vi "Visible_Ch_Init.vi"   [LabVIEW 2017]
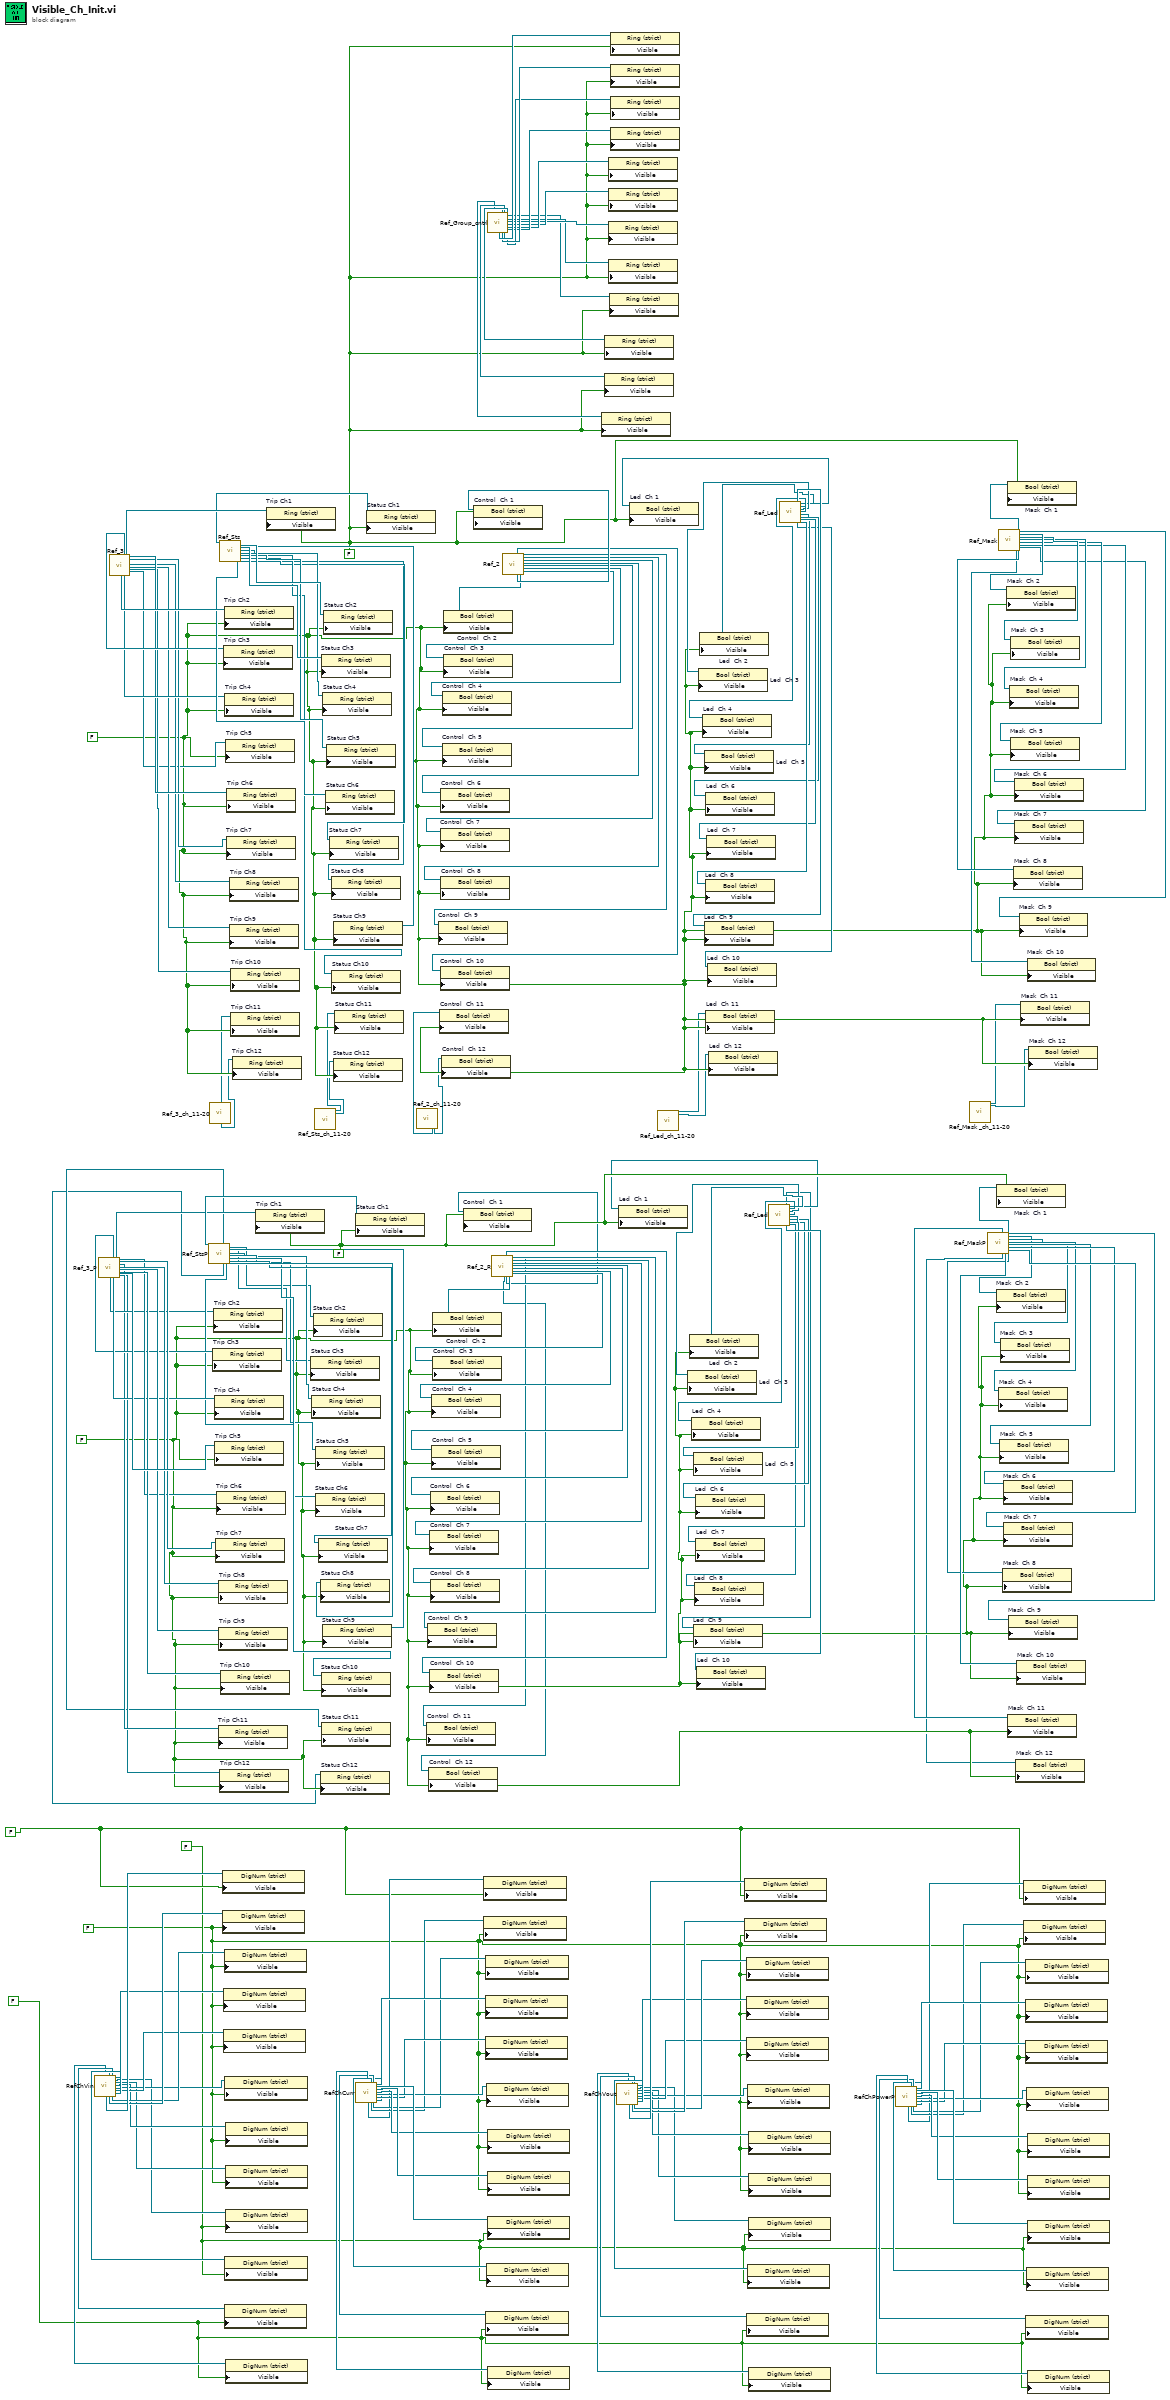
[diagram p0: block diagram]
diagram:
  w14 = FALSE
  w15 = FALSE
  w16 = FALSE
  w17 = FALSE
  w82 = FALSE
  w126 = FALSE
  w76 = FALSE
  w1 = FALSE
  n1 = call "RefChVin.vi"() -> ("Vin  P1 out"=w65:refnum<vi>, "Vin  P12 out"=w54:refnum<vi>, "Vin  P2 out"=w64:refnum<vi>, "Vin  P11 out"=w55:refnum<vi>, "Vin  P3 out"=w63:refnum<vi>, "Vin  P10 out"=w56:refnum<vi>, "Vin  P9 out"=w57:refnum<vi>, "Vin  P8 out"=w58:refnum<vi>, "Vin  P7 out"=w59:refnum<vi>, "Vin  P6 out"=w60:refnum<vi>, "Vin  P5 out"=w61:refnum<vi>, "Vin  P4 out"=w62:refnum<vi>)  [unwired: 15 in, 1 out]
  n2 = call "Ref_3_P.vi"() -> ("Trip  Ch 1 out"=w86:refnum<vi>, "Trip  Ch 2 out"=w89:refnum<vi>, "Trip  Ch 3 out"=w105:refnum<vi>, "Trip  Ch 4 out"=w106:refnum<vi>, "Trip  Ch 5 out"=w125:refnum<vi>, "Trip  Ch 6 out"=w107:refnum<vi>, "Trip  Ch 7 out"=w108:refnum<vi>, "Trip  Ch 11 out"=w85:refnum<vi>, "Trip  Ch 8 out"=w109:refnum<vi>, "Trip  Ch 9 out"=w110:refnum<vi>, "Trip  Ch 10 out"=w111:refnum<vi>, "Trip  Ch 12 out"=w84:refnum<vi>)  [unwired: 16 in]
  n3 = call "Ref_3.vi"() -> ("Trip  Ch 1 out"=w186:refnum<vi>, "Trip  Ch 2 out"=w183:refnum<vi>, "Trip  Ch 3 out"=w167:refnum<vi>, "Trip  Ch 4 out"=w166:refnum<vi>, "Trip  Ch 5 out"=w147:refnum<vi>, "Trip  Ch 6 out"=w165:refnum<vi>, "Trip  Ch 7 out"=w164:refnum<vi>, "Trip  Ch 8 out"=w163:refnum<vi>, "Trip  Ch 9 out"=w162:refnum<vi>, "Trip  Ch 10 out"=w161:refnum<vi>)  [unwired: 18 in]
  n4 = call "Ref_StsP.vi"() -> ("Status Ch11 out"=w83:refnum<vi>, "Status Ch12 out"=w81:refnum<vi>, "Status Ch9 out"=w103:refnum<vi>, "Status Ch10 out"=w104:refnum<vi>, "Status Ch1 out"=w87:refnum<vi>, "Status Ch2 out"=w97:refnum<vi>, "Status Ch3 out"=w98:refnum<vi>, "Status Ch4 out"=w99:refnum<vi>, "Status Ch5 out"=w100:refnum<vi>, "Status Ch6 out"=w101:refnum<vi>, "Status Ch7 out"=w102:refnum<vi>, "Status Ch8 out"=w114:refnum<vi>)  [unwired: 16 in]
  n5 = call "Ref_3_ch_11-20.vi"() -> ("Trip  Ch 11 out"=w75:refnum<vi>, "Trip  Ch 12 out"=w74:refnum<vi>)  [unwired: 18 in, 8 out]
  n6 = property on="Trip Ch3" class="Ring (strict)"(reference=w105, "Visible"=w82) -> ()  [unwired: 1 in, 2 out]
  n7 = property on="Trip Ch2" class="Ring (strict)"(reference=w89, "Visible"=w82) -> ()  [unwired: 1 in, 2 out]
  n8 = property on="Trip Ch4" class="Ring (strict)"(reference=w106, "Visible"=w82) -> ()  [unwired: 1 in, 2 out]
  n9 = property on="Trip Ch5" class="Ring (strict)"(reference=w125, "Visible"=w82) -> ()  [unwired: 1 in, 2 out]
  n10 = property on="Trip Ch7" class="Ring (strict)"(reference=w108, "Visible"=w82) -> ()  [unwired: 1 in, 2 out]
  n11 = property on="Trip Ch6" class="Ring (strict)"(reference=w107, "Visible"=w82) -> ()  [unwired: 1 in, 2 out]
  n12 = property on="Trip Ch11" class="Ring (strict)"(reference=w85, "Visible"=w82) -> ()  [unwired: 1 in, 2 out]
  n13 = property on="Trip Ch8" class="Ring (strict)"(reference=w109, "Visible"=w82) -> ()  [unwired: 1 in, 2 out]
  n14 = property on="Trip Ch9" class="Ring (strict)"(reference=w110, "Visible"=w82) -> ()  [unwired: 1 in, 2 out]
  n15 = call "Ref_Sts.vi"() -> ("Status Ch9 out"=w169:refnum<vi>, "Status Ch10 out"=w168:refnum<vi>, "Status Ch1 out"=w185:refnum<vi>, "Status Ch2 out"=w175:refnum<vi>, "Status Ch3 out"=w174:refnum<vi>, "Status Ch4 out"=w173:refnum<vi>, "Status Ch5 out"=w172:refnum<vi>, "Status Ch6 out"=w171:refnum<vi>, "Status Ch7 out"=w170:refnum<vi>, "Status Ch8 out"=w158:refnum<vi>)  [unwired: 18 in]
  n16 = property on="Trip Ch12" class="Ring (strict)"(reference=w84, "Visible"=w82) -> ()  [unwired: 1 in, 2 out]
  n17 = property on="Trip Ch10" class="Ring (strict)"(reference=w111, "Visible"=w82) -> ()  [unwired: 1 in, 2 out]
  n18 = property class="DigNum (strict)"(reference=w65, "Visible"=w16) -> ()  [unwired: 1 in, 2 out]
  n19 = property class="DigNum (strict)"(reference=w64, "Visible"=w14) -> ()  [unwired: 1 in, 2 out]
  n20 = property on="Trip Ch3" class="Ring (strict)"(reference=w167, "Visible"=w76) -> ()  [unwired: 1 in, 2 out]
  n21 = property class="DigNum (strict)"(reference=w62, "Visible"=w14) -> ()  [unwired: 1 in, 2 out]
  n22 = property class="DigNum (strict)"(reference=w61, "Visible"=w14) -> ()  [unwired: 1 in, 2 out]
  n23 = property on="Trip Ch2" class="Ring (strict)"(reference=w183, "Visible"=w76) -> ()  [unwired: 1 in, 2 out]
  n24 = property class="DigNum (strict)"(reference=w63, "Visible"=w14) -> ()  [unwired: 1 in, 2 out]
  n25 = property class="DigNum (strict)"(reference=w55, "Visible"=w17) -> ()  [unwired: 1 in, 2 out]
  n26 = property on="Trip Ch4" class="Ring (strict)"(reference=w166, "Visible"=w76) -> ()  [unwired: 1 in, 2 out]
  n27 = property class="DigNum (strict)"(reference=w60, "Visible"=w14) -> ()  [unwired: 1 in, 2 out]
  n28 = property class="DigNum (strict)"(reference=w56, "Visible"=w15) -> ()  [unwired: 1 in, 2 out]
  n29 = property on="Trip Ch5" class="Ring (strict)"(reference=w147, "Visible"=w76) -> ()  [unwired: 1 in, 2 out]
  n30 = property class="DigNum (strict)"(reference=w59, "Visible"=w14) -> ()  [unwired: 1 in, 2 out]
  n31 = property class="DigNum (strict)"(reference=w58, "Visible"=w14) -> ()  [unwired: 1 in, 2 out]
  n32 = property class="DigNum (strict)"(reference=w57, "Visible"=w15) -> ()  [unwired: 1 in, 2 out]
  n33 = property class="DigNum (strict)"(reference=w54, "Visible"=w17) -> ()  [unwired: 1 in, 2 out]
  n34 = property on="Trip Ch7" class="Ring (strict)"(reference=w164, "Visible"=w76) -> ()  [unwired: 1 in, 2 out]
  n35 = property on="Trip Ch6" class="Ring (strict)"(reference=w165, "Visible"=w76) -> ()  [unwired: 1 in, 2 out]
  n36 = property on="Trip Ch8" class="Ring (strict)"(reference=w163, "Visible"=w76) -> ()  [unwired: 1 in, 2 out]
  n37 = property on="Trip Ch9" class="Ring (strict)"(reference=w162, "Visible"=w76) -> ()  [unwired: 1 in, 2 out]
  n38 = property on="Trip Ch10" class="Ring (strict)"(reference=w161, "Visible"=w76) -> ()  [unwired: 1 in, 2 out]
  n39 = property on="Trip Ch11" class="Ring (strict)"(reference=w75, "Visible"=w76) -> ()  [unwired: 1 in, 2 out]
  n40 = property on="Trip Ch12" class="Ring (strict)"(reference=w74, "Visible"=w76) -> ()  [unwired: 1 in, 2 out]
  n41 = property on="Trip Ch1" class="Ring (strict)"(reference=w86, "Visible"=w126) -> ()  [unwired: 1 in, 2 out]
  n42 = property on="Trip Ch1" class="Ring (strict)"(reference=w186, "Visible"=w1) -> ()  [unwired: 1 in, 2 out]
  n43 = property on="Status Ch3" class="Ring (strict)"(reference=w98, "Visible"=w82) -> ()  [unwired: 1 in, 2 out]
  n44 = property on="Status Ch4" class="Ring (strict)"(reference=w99, "Visible"=w82) -> ()  [unwired: 1 in, 2 out]
  n45 = property on="Status Ch2" class="Ring (strict)"(reference=w97, "Visible"=w82) -> ()  [unwired: 1 in, 2 out]
  n46 = call "Ref_Sts_ch_11-20.vi"() -> ("Status Ch 11 out"=w73:refnum<vi>, "Status Ch 12 out"=w72:refnum<vi>)  [unwired: 18 in, 8 out]
  n47 = property on="Status Ch6" class="Ring (strict)"(reference=w101, "Visible"=w82) -> ()  [unwired: 1 in, 2 out]
  n48 = property on="Status Ch5" class="Ring (strict)"(reference=w100, "Visible"=w82) -> ()  [unwired: 1 in, 2 out]
  n49 = property on="Status Ch7" class="Ring (strict)"(reference=w102, "Visible"=w82) -> ()  [unwired: 1 in, 2 out]
  n50 = property on="Status Ch8" class="Ring (strict)"(reference=w114, "Visible"=w82) -> ()  [unwired: 1 in, 2 out]
  n51 = property on="Status Ch12" class="Ring (strict)"(reference=w81, "Visible"=w82) -> ()  [unwired: 1 in, 2 out]
  n52 = property on="Status Ch3" class="Ring (strict)"(reference=w174, "Visible"=w76) -> ()  [unwired: 1 in, 2 out]
  n53 = property on="Status Ch10" class="Ring (strict)"(reference=w104, "Visible"=w82) -> ()  [unwired: 1 in, 2 out]
  n54 = property on="Status Ch11" class="Ring (strict)"(reference=w83, "Visible"=w82) -> ()  [unwired: 1 in, 2 out]
  n55 = property on="Status Ch4" class="Ring (strict)"(reference=w173, "Visible"=w76) -> ()  [unwired: 1 in, 2 out]
  n56 = property on="Status Ch9" class="Ring (strict)"(reference=w103, "Visible"=w82) -> ()  [unwired: 1 in, 2 out]
  n57 = property on="Status Ch2" class="Ring (strict)"(reference=w175, "Visible"=w76) -> ()  [unwired: 1 in, 2 out]
  n58 = property on="Status Ch6" class="Ring (strict)"(reference=w171, "Visible"=w76) -> ()  [unwired: 1 in, 2 out]
  n59 = property on="Status Ch5" class="Ring (strict)"(reference=w172, "Visible"=w76) -> ()  [unwired: 1 in, 2 out]
  n60 = property on="Status Ch7" class="Ring (strict)"(reference=w170, "Visible"=w76) -> ()  [unwired: 1 in, 2 out]
  n61 = property on="Status Ch8" class="Ring (strict)"(reference=w158, "Visible"=w76) -> ()  [unwired: 1 in, 2 out]
  n62 = property on="Status Ch10" class="Ring (strict)"(reference=w168, "Visible"=w76) -> ()  [unwired: 1 in, 2 out]
  n63 = property on="Status Ch9" class="Ring (strict)"(reference=w169, "Visible"=w76) -> ()  [unwired: 1 in, 2 out]
  n64 = property on="Status Ch12" class="Ring (strict)"(reference=w72, "Visible"=w76) -> ()  [unwired: 1 in, 2 out]
  n65 = property on="Status Ch11" class="Ring (strict)"(reference=w73, "Visible"=w76) -> ()  [unwired: 1 in, 2 out]
  n66 = property on="Status Ch1" class="Ring (strict)"(reference=w87, "Visible"=w126) -> ()  [unwired: 1 in, 2 out]
  n67 = call "RefChCurr.vi"() -> ("Current P1 out"=w42:refnum<vi>, "Current P12 out"=w53:refnum<vi>, "Current P2 out"=w43:refnum<vi>, "Current P11 out"=w52:refnum<vi>, "Current P3 out"=w44:refnum<vi>, "Current P10 out"=w51:refnum<vi>, "Current P9 out"=w50:refnum<vi>, "Current P8 out"=w49:refnum<vi>, "Current P7 out"=w48:refnum<vi>, "Current P6 out"=w47:refnum<vi>, "Current P5 out"=w46:refnum<vi>, "Current P4 out"=w45:refnum<vi>)  [unwired: 15 in, 1 out]
  n68 = property on="Status Ch1" class="Ring (strict)"(reference=w185, "Visible"=w1) -> ()  [unwired: 1 in, 2 out]
  n69 = call "Ref_2_ch_11-20.vi"() -> ("Control  Ch 11 out"=w71:refnum<vi>, "Control  Ch 12 out"=w70:refnum<vi>)  [unwired: 17 in, 9 out]
  n70 = property on="Control  Ch 11" class="Bool (strict)"(reference=w71, "Visible"=w76) -> ()  [unwired: 1 in, 2 out]
  n71 = property on="Control  Ch 12" class="Bool (strict)"(reference=w70, "Visible"=w76) -> ()  [unwired: 1 in, 2 out]
  n72 = property class="DigNum (strict)"(reference=w42, "Visible"=w16) -> ()  [unwired: 1 in, 2 out]
  n73 = property class="DigNum (strict)"(reference=w43, "Visible"=w14) -> ()  [unwired: 1 in, 2 out]
  n74 = property class="DigNum (strict)"(reference=w45, "Visible"=w14) -> ()  [unwired: 1 in, 2 out]
  n75 = property class="DigNum (strict)"(reference=w46, "Visible"=w14) -> ()  [unwired: 1 in, 2 out]
  n76 = property class="DigNum (strict)"(reference=w44, "Visible"=w14) -> ()  [unwired: 1 in, 2 out]
  n77 = property class="DigNum (strict)"(reference=w52, "Visible"=w17) -> ()  [unwired: 1 in, 2 out]
  n78 = property class="DigNum (strict)"(reference=w47, "Visible"=w14) -> ()  [unwired: 1 in, 2 out]
  n79 = property class="DigNum (strict)"(reference=w51, "Visible"=w15) -> ()  [unwired: 1 in, 2 out]
  n80 = call "Ref_Group_cntrl.vi"() -> ("Group ch 1 out"=w13:refnum<vi>, "Group ch 12 out"=w2:refnum<vi>, "Group ch 2 out"=w12:refnum<vi>, "Group ch 11 out"=w3:refnum<vi>, "Group ch 3 out"=w11:refnum<vi>, "Group ch 10 out"=w4:refnum<vi>, "Group ch 9 out"=w5:refnum<vi>, "Group ch 8 out"=w6:refnum<vi>, "Group ch 7 out"=w7:refnum<vi>, "Group ch 6 out"=w8:refnum<vi>, "Group ch 5 out"=w9:refnum<vi>, "Group ch 4 out"=w10:refnum<vi>)  [unwired: 15 in, 1 out]
  n81 = property class="DigNum (strict)"(reference=w48, "Visible"=w14) -> ()  [unwired: 1 in, 2 out]
  n82 = property class="DigNum (strict)"(reference=w49, "Visible"=w14) -> ()  [unwired: 1 in, 2 out]
  n83 = property class="DigNum (strict)"(reference=w50, "Visible"=w15) -> ()  [unwired: 1 in, 2 out]
  n84 = property class="DigNum (strict)"(reference=w53, "Visible"=w17) -> ()  [unwired: 1 in, 2 out]
  n85 = call "Ref_2_R.vi"() -> ("Control  Ch 12 out"=w79:refnum<vi>, "Control  Ch 10 out"=w96:refnum<vi>, "Control  Ch 1 out"=w88:refnum<vi>, "Control  Ch 9 out"=w95:refnum<vi>, "Control  Ch 2 out"=w90:refnum<vi>, "Control  Ch 11 out"=w80:refnum<vi>, "Control  Ch 8 out"=w94:refnum<vi>, "Control  Ch 7 out"=w93:refnum<vi>, "Control  Ch 6 out"=w113:refnum<vi>, "Control  Ch 5 out"=w92:refnum<vi>, "Control  Ch 4 out"=w91:refnum<vi>, "Control  Ch 3 out"=w112:refnum<vi>)  [unwired: 15 in, 1 out]
  n86 = property on="Control  Ch 11" class="Bool (strict)"(reference=w80, "Visible"=w82) -> ()  [unwired: 1 in, 2 out]
  n87 = property on="Control  Ch 9" class="Bool (strict)"(reference=w95, "Visible"=w82) -> ()  [unwired: 1 in, 2 out]
  n88 = property on="Control  Ch 12" class="Bool (strict)"(reference=w79, "Visible"=w82) -> ()  [unwired: 1 in, 2 out]
  n89 = property on="Control  Ch 7" class="Bool (strict)"(reference=w93, "Visible"=w82) -> ()  [unwired: 1 in, 2 out]
  n90 = property on="Control  Ch 10" class="Bool (strict)"(reference=w96, "Visible"=w82) -> ()  [unwired: 1 in, 2 out]
  n91 = property on="Control  Ch 6" class="Bool (strict)"(reference=w113, "Visible"=w82) -> ()  [unwired: 1 in, 2 out]
  n92 = property on="Control  Ch 8" class="Bool (strict)"(reference=w94, "Visible"=w82) -> ()  [unwired: 1 in, 2 out]
  n93 = property on="Control  Ch 4" class="Bool (strict)"(reference=w91, "Visible"=w82) -> ()  [unwired: 1 in, 2 out]
  n94 = property on="Control  Ch 5" class="Bool (strict)"(reference=w92, "Visible"=w82) -> ()  [unwired: 1 in, 2 out]
  n95 = property on="Control  Ch 2" class="Bool (strict)"(reference=w90, "Visible"=w82) -> ()  [unwired: 1 in, 2 out]
  n96 = property on="Control  Ch 3" class="Bool (strict)"(reference=w112, "Visible"=w82) -> ()  [unwired: 1 in, 2 out]
  n97 = property on="Control  Ch 1" class="Bool (strict)"(reference=w88, "Visible"=w126) -> ()  [unwired: 1 in, 2 out]
  n98 = call "Ref_2.vi"() -> ("Control  Ch 10 out"=w176:refnum<vi>, "Control  Ch 1 out"=w184:refnum<vi>, "Control  Ch 9 out"=w177:refnum<vi>, "Control  Ch 2 out"=w182:refnum<vi>, "Control  Ch 8 out"=w178:refnum<vi>, "Control  Ch 7 out"=w179:refnum<vi>, "Control  Ch 6 out"=w159:refnum<vi>, "Control  Ch 5 out"=w180:refnum<vi>, "Control  Ch 4 out"=w181:refnum<vi>, "Control  Ch 3 out"=w160:refnum<vi>)  [unwired: 17 in, 1 out]
  n99 = property on="Control  Ch 9" class="Bool (strict)"(reference=w177, "Visible"=w76) -> ()  [unwired: 1 in, 2 out]
  n100 = property on="Control  Ch 7" class="Bool (strict)"(reference=w179, "Visible"=w76) -> ()  [unwired: 1 in, 2 out]
  n101 = property on="Control  Ch 10" class="Bool (strict)"(reference=w176, "Visible"=w76) -> ()  [unwired: 1 in, 2 out]
  n102 = property on="Control  Ch 6" class="Bool (strict)"(reference=w159, "Visible"=w76) -> ()  [unwired: 1 in, 2 out]
  n103 = property on="Control  Ch 8" class="Bool (strict)"(reference=w178, "Visible"=w76) -> ()  [unwired: 1 in, 2 out]
  n104 = property on="Control  Ch 4" class="Bool (strict)"(reference=w181, "Visible"=w76) -> ()  [unwired: 1 in, 2 out]
  n105 = property on="Control  Ch 5" class="Bool (strict)"(reference=w180, "Visible"=w76) -> ()  [unwired: 1 in, 2 out]
  n106 = property on="Control  Ch 2" class="Bool (strict)"(reference=w182, "Visible"=w76) -> ()  [unwired: 1 in, 2 out]
  n107 = property on="Control  Ch 3" class="Bool (strict)"(reference=w160, "Visible"=w76) -> ()  [unwired: 1 in, 2 out]
  n108 = property on="Control  Ch 1" class="Bool (strict)"(reference=w184, "Visible"=w1) -> ()  [unwired: 1 in, 2 out]
  n109 = property class="Ring (strict)"(reference=w2, "Visible"=w1) -> ()  [unwired: 1 in, 2 out]
  n110 = property class="Ring (strict)"(reference=w3, "Visible"=w1) -> ()  [unwired: 1 in, 2 out]
  n111 = property class="Ring (strict)"(reference=w4, "Visible"=w1) -> ()  [unwired: 1 in, 2 out]
  n112 = property class="Ring (strict)"(reference=w7, "Visible"=w1) -> ()  [unwired: 1 in, 2 out]
  n113 = property class="Ring (strict)"(reference=w9, "Visible"=w1) -> ()  [unwired: 1 in, 2 out]
  n114 = property class="Ring (strict)"(reference=w8, "Visible"=w1) -> ()  [unwired: 1 in, 2 out]
  n115 = property class="Ring (strict)"(reference=w6, "Visible"=w1) -> ()  [unwired: 1 in, 2 out]
  n116 = property class="Ring (strict)"(reference=w5, "Visible"=w1) -> ()  [unwired: 1 in, 2 out]
  n117 = property class="Ring (strict)"(reference=w12, "Visible"=w1) -> ()  [unwired: 1 in, 2 out]
  n118 = property class="Ring (strict)"(reference=w10, "Visible"=w1) -> ()  [unwired: 1 in, 2 out]
  n119 = property class="Ring (strict)"(reference=w13, "Visible"=w1) -> ()  [unwired: 1 in, 2 out]
  n120 = property class="Ring (strict)"(reference=w11, "Visible"=w1) -> ()  [unwired: 1 in, 2 out]
  n121 = call "RefChVout.vi"() -> ("Vout  P1 out"=w41:refnum<vi>, "Vout  P12 out"=w30:refnum<vi>, "Vout  P2 out"=w40:refnum<vi>, "Vout  P11 out"=w31:refnum<vi>, "Vout  P3 out"=w39:refnum<vi>, "Vout  P10 out"=w32:refnum<vi>, "Vout  P9 out"=w33:refnum<vi>, "Vout  P8 out"=w34:refnum<vi>, "Vout  P7 out"=w35:refnum<vi>, "Vout  P6 out"=w36:refnum<vi>, "Vout  P5 out"=w37:refnum<vi>, "Vout  P4 out"=w38:refnum<vi>)  [unwired: 15 in, 1 out]
  n122 = call "Ref_Led_ch_11-20.vi"() -> ("Led Ch 11 out"=w69:refnum<vi>, "Led Ch 12 out"=w68:refnum<vi>)  [unwired: 18 in, 8 out]
  n123 = property on="Led  Ch 11" class="Bool (strict)"(reference=w69, "Visible"=w76) -> ()  [unwired: 1 in, 2 out]
  n124 = property on="Led  Ch 12" class="Bool (strict)"(reference=w68, "Visible"=w76) -> ()  [unwired: 1 in, 2 out]
  n125 = property class="DigNum (strict)"(reference=w41, "Visible"=w16) -> ()  [unwired: 1 in, 2 out]
  n126 = property class="DigNum (strict)"(reference=w40, "Visible"=w14) -> ()  [unwired: 1 in, 2 out]
  n127 = property class="DigNum (strict)"(reference=w38, "Visible"=w14) -> ()  [unwired: 1 in, 2 out]
  n128 = property class="DigNum (strict)"(reference=w37, "Visible"=w14) -> ()  [unwired: 1 in, 2 out]
  n129 = property class="DigNum (strict)"(reference=w39, "Visible"=w14) -> ()  [unwired: 1 in, 2 out]
  n130 = property class="DigNum (strict)"(reference=w31, "Visible"=w17) -> ()  [unwired: 1 in, 2 out]
  n131 = property class="DigNum (strict)"(reference=w36, "Visible"=w14) -> ()  [unwired: 1 in, 2 out]
  n132 = property class="DigNum (strict)"(reference=w32, "Visible"=w15) -> ()  [unwired: 1 in, 2 out]
  n133 = property class="DigNum (strict)"(reference=w35, "Visible"=w14) -> ()  [unwired: 1 in, 2 out]
  n134 = property class="DigNum (strict)"(reference=w34, "Visible"=w14) -> ()  [unwired: 1 in, 2 out]
  n135 = property class="DigNum (strict)"(reference=w33, "Visible"=w15) -> ()  [unwired: 1 in, 2 out]
  n136 = property class="DigNum (strict)"(reference=w30, "Visible"=w17) -> ()  [unwired: 1 in, 2 out]
  n137 = call "Ref_Led.vi"() -> ("Led Ch 9 out"=w115:refnum<vi>, "Led Ch 10 out"=w122:refnum<vi>, "Led Ch 1 out"=w123:refnum<vi>, "Led Ch 2 out"=w124:refnum<vi>, "Led Ch 3 out"=w121:refnum<vi>, "Led Ch 4 out"=w120:refnum<vi>, "Led Ch 5 out"=w119:refnum<vi>, "Led Ch 6 out"=w118:refnum<vi>, "Led Ch 7 out"=w117:refnum<vi>, "Led Ch 8 out"=w116:refnum<vi>)  [unwired: 18 in]
  n138 = property on="Led  Ch 1" class="Bool (strict)"(reference=w123, "Visible"=w126) -> ()  [unwired: 1 in, 2 out]
  n139 = property on="Led  Ch 3" class="Bool (strict)"(reference=w121, "Visible"=w82) -> ()  [unwired: 1 in, 2 out]
  n140 = property on="Led  Ch 2" class="Bool (strict)"(reference=w124, "Visible"=w82) -> ()  [unwired: 1 in, 2 out]
  n141 = property on="Led  Ch 4" class="Bool (strict)"(reference=w120, "Visible"=w82) -> ()  [unwired: 1 in, 2 out]
  n142 = property on="Led  Ch 5" class="Bool (strict)"(reference=w119, "Visible"=w82) -> ()  [unwired: 1 in, 2 out]
  n143 = property on="Led  Ch 9" class="Bool (strict)"(reference=w115, "Visible"=w82) -> ()  [unwired: 1 in, 2 out]
  n144 = property on="Led  Ch 8" class="Bool (strict)"(reference=w116, "Visible"=w82) -> ()  [unwired: 1 in, 2 out]
  n145 = property on="Led  Ch 6" class="Bool (strict)"(reference=w118, "Visible"=w82) -> ()  [unwired: 1 in, 2 out]
  n146 = property on="Led  Ch 7" class="Bool (strict)"(reference=w117, "Visible"=w82) -> ()  [unwired: 1 in, 2 out]
  n147 = property on="Led  Ch 10" class="Bool (strict)"(reference=w122, "Visible"=w82) -> ()  [unwired: 1 in, 2 out]
  n148 = call "Ref_Led.vi"() -> ("Led Ch 9 out"=w157:refnum<vi>, "Led Ch 10 out"=w150:refnum<vi>, "Led Ch 1 out"=w149:refnum<vi>, "Led Ch 2 out"=w148:refnum<vi>, "Led Ch 3 out"=w151:refnum<vi>, "Led Ch 4 out"=w152:refnum<vi>, "Led Ch 5 out"=w153:refnum<vi>, "Led Ch 6 out"=w154:refnum<vi>, "Led Ch 7 out"=w155:refnum<vi>, "Led Ch 8 out"=w156:refnum<vi>)  [unwired: 18 in]
  n149 = property on="Led  Ch 1" class="Bool (strict)"(reference=w149, "Visible"=w1) -> ()  [unwired: 1 in, 2 out]
  n150 = property on="Led  Ch 3" class="Bool (strict)"(reference=w151, "Visible"=w76) -> ()  [unwired: 1 in, 2 out]
  n151 = property on="Led  Ch 2" class="Bool (strict)"(reference=w148, "Visible"=w76) -> ()  [unwired: 1 in, 2 out]
  n152 = property on="Led  Ch 4" class="Bool (strict)"(reference=w152, "Visible"=w76) -> ()  [unwired: 1 in, 2 out]
  n153 = property on="Led  Ch 5" class="Bool (strict)"(reference=w153, "Visible"=w76) -> ()  [unwired: 1 in, 2 out]
  n154 = property on="Led  Ch 9" class="Bool (strict)"(reference=w157, "Visible"=w76) -> ()  [unwired: 1 in, 2 out]
  n155 = property on="Led  Ch 8" class="Bool (strict)"(reference=w156, "Visible"=w76) -> ()  [unwired: 1 in, 2 out]
  n156 = property on="Led  Ch 6" class="Bool (strict)"(reference=w154, "Visible"=w76) -> ()  [unwired: 1 in, 2 out]
  n157 = property on="Led  Ch 7" class="Bool (strict)"(reference=w155, "Visible"=w76) -> ()  [unwired: 1 in, 2 out]
  n158 = property on="Led  Ch 10" class="Bool (strict)"(reference=w150, "Visible"=w76) -> ()  [unwired: 1 in, 2 out]
  n159 = call "RefChPowerP.vi"() -> ("Pwr  P1 out"=w18:refnum<vi>, "Pwr  P12 out"=w29:refnum<vi>, "Pwr  P2 out"=w19:refnum<vi>, "Pwr  P11 out"=w28:refnum<vi>, "Pwr  P3 out"=w20:refnum<vi>, "Pwr  P10 out"=w27:refnum<vi>, "Pwr  P9 out"=w26:refnum<vi>, "Pwr  P8 out"=w25:refnum<vi>, "Pwr  P7 out"=w24:refnum<vi>, "Pwr  P6 out"=w23:refnum<vi>, "Pwr  P5 out"=w22:refnum<vi>, "Pwr  P4 out"=w21:refnum<vi>)  [unwired: 15 in, 1 out]
  n160 = call "Ref_Mask _ch_11-20.vi"() -> ("Mask Ch 11 out"=w67:refnum<vi>, "Mask Ch 12 out"=w66:refnum<vi>)  [unwired: 18 in, 8 out]
  n161 = call "Ref_MaskP.vi"() -> ("Mask Ch 11 out"=w78:refnum<vi>, "Mask Ch 12 out"=w77:refnum<vi>, "Mask Ch 9 out"=w136:refnum<vi>, "Mask Ch 10 out"=w134:refnum<vi>, "Mask Ch 1 out"=w135:refnum<vi>, "Mask Ch 2 out"=w127:refnum<vi>, "Mask Ch 3 out"=w128:refnum<vi>, "Mask Ch 4 out"=w129:refnum<vi>, "Mask Ch 5 out"=w130:refnum<vi>, "Mask Ch 6 out"=w131:refnum<vi>, "Mask Ch 7 out"=w132:refnum<vi>, "Mask Ch 8 out"=w133:refnum<vi>)  [unwired: 16 in]
  n162 = property on="Mask  Ch 2" class="Bool (strict)"(reference=w127, "Visible"=w82) -> ()  [unwired: 1 in, 2 out]
  n163 = property on="Mask  Ch 1" class="Bool (strict)"(reference=w135, "Visible"=w126) -> ()  [unwired: 1 in, 2 out]
  n164 = call "Ref_Mask.vi"() -> ("Mask Ch 9 out"=w137:refnum<vi>, "Mask Ch 10 out"=w139:refnum<vi>, "Mask Ch 1 out"=w138:refnum<vi>, "Mask Ch 2 out"=w146:refnum<vi>, "Mask Ch 3 out"=w145:refnum<vi>, "Mask Ch 4 out"=w144:refnum<vi>, "Mask Ch 5 out"=w143:refnum<vi>, "Mask Ch 6 out"=w142:refnum<vi>, "Mask Ch 7 out"=w141:refnum<vi>, "Mask Ch 8 out"=w140:refnum<vi>)  [unwired: 18 in]
  n165 = property on="Mask  Ch 4" class="Bool (strict)"(reference=w129, "Visible"=w82) -> ()  [unwired: 1 in, 2 out]
  n166 = property on="Mask  Ch 5" class="Bool (strict)"(reference=w130, "Visible"=w82) -> ()  [unwired: 1 in, 2 out]
  n167 = property on="Mask  Ch 3" class="Bool (strict)"(reference=w128, "Visible"=w82) -> ()  [unwired: 1 in, 2 out]
  n168 = property on="Mask  Ch 8" class="Bool (strict)"(reference=w133, "Visible"=w82) -> ()  [unwired: 1 in, 2 out]
  n169 = property on="Mask  Ch 6" class="Bool (strict)"(reference=w131, "Visible"=w82) -> ()  [unwired: 1 in, 2 out]
  n170 = property on="Mask  Ch 7" class="Bool (strict)"(reference=w132, "Visible"=w82) -> ()  [unwired: 1 in, 2 out]
  n171 = property on="Mask  Ch 2" class="Bool (strict)"(reference=w146, "Visible"=w76) -> ()  [unwired: 1 in, 2 out]
  n172 = property on="Mask  Ch 1" class="Bool (strict)"(reference=w138, "Visible"=w1) -> ()  [unwired: 1 in, 2 out]
  n173 = property on="Mask  Ch 11" class="Bool (strict)"(reference=w78, "Visible"=w82) -> ()  [unwired: 1 in, 2 out]
  n174 = property on="Mask  Ch 9" class="Bool (strict)"(reference=w136, "Visible"=w82) -> ()  [unwired: 1 in, 2 out]
  n175 = property on="Mask  Ch 4" class="Bool (strict)"(reference=w144, "Visible"=w76) -> ()  [unwired: 1 in, 2 out]
  n176 = property on="Mask  Ch 5" class="Bool (strict)"(reference=w143, "Visible"=w76) -> ()  [unwired: 1 in, 2 out]
  n177 = property on="Mask  Ch 3" class="Bool (strict)"(reference=w145, "Visible"=w76) -> ()  [unwired: 1 in, 2 out]
  n178 = property on="Mask  Ch 8" class="Bool (strict)"(reference=w140, "Visible"=w76) -> ()  [unwired: 1 in, 2 out]
  n179 = property on="Mask  Ch 6" class="Bool (strict)"(reference=w142, "Visible"=w76) -> ()  [unwired: 1 in, 2 out]
  n180 = property on="Mask  Ch 7" class="Bool (strict)"(reference=w141, "Visible"=w76) -> ()  [unwired: 1 in, 2 out]
  n181 = property on="Mask  Ch 12" class="Bool (strict)"(reference=w77, "Visible"=w82) -> ()  [unwired: 1 in, 2 out]
  n182 = property on="Mask  Ch 10" class="Bool (strict)"(reference=w134, "Visible"=w82) -> ()  [unwired: 1 in, 2 out]
  n183 = property on="Mask  Ch 9" class="Bool (strict)"(reference=w137, "Visible"=w76) -> ()  [unwired: 1 in, 2 out]
  n184 = property on="Mask  Ch 11" class="Bool (strict)"(reference=w67, "Visible"=w76) -> ()  [unwired: 1 in, 2 out]
  n185 = property class="DigNum (strict)"(reference=w18, "Visible"=w16) -> ()  [unwired: 1 in, 2 out]
  n186 = property class="DigNum (strict)"(reference=w19, "Visible"=w14) -> ()  [unwired: 1 in, 2 out]
  n187 = property class="DigNum (strict)"(reference=w21, "Visible"=w14) -> ()  [unwired: 1 in, 2 out]
  n188 = property class="DigNum (strict)"(reference=w22, "Visible"=w14) -> ()  [unwired: 1 in, 2 out]
  n189 = property class="DigNum (strict)"(reference=w20, "Visible"=w14) -> ()  [unwired: 1 in, 2 out]
  n190 = property class="DigNum (strict)"(reference=w28, "Visible"=w17) -> ()  [unwired: 1 in, 2 out]
  n191 = property class="DigNum (strict)"(reference=w23, "Visible"=w14) -> ()  [unwired: 1 in, 2 out]
  n192 = property class="DigNum (strict)"(reference=w27, "Visible"=w15) -> ()  [unwired: 1 in, 2 out]
  n193 = property on="Mask  Ch 10" class="Bool (strict)"(reference=w139, "Visible"=w76) -> ()  [unwired: 1 in, 2 out]
  n194 = property class="DigNum (strict)"(reference=w24, "Visible"=w14) -> ()  [unwired: 1 in, 2 out]
  n195 = property class="DigNum (strict)"(reference=w25, "Visible"=w14) -> ()  [unwired: 1 in, 2 out]
  n196 = property class="DigNum (strict)"(reference=w26, "Visible"=w15) -> ()  [unwired: 1 in, 2 out]
  n197 = property class="DigNum (strict)"(reference=w29, "Visible"=w17) -> ()  [unwired: 1 in, 2 out]
  n198 = property on="Mask  Ch 12" class="Bool (strict)"(reference=w66, "Visible"=w76) -> ()  [unwired: 1 in, 2 out]
